vi "Wire RefNum to BBN.vi"(8 "error in (no error)":errorcluster, 9 "Label.Text":string, 10 "Created RefNum":refnum<vi>, 11 "VI in":refnum<vi>) -> (0 "error out":errorcluster)   [LabVIEW 2020]
uses:
  <vilib>/Utility/traverseref.llb/TRef TravTarget.ctl
  <vilib>/Utility/traverseref.llb/VI Scripting - Traverse.lvlib
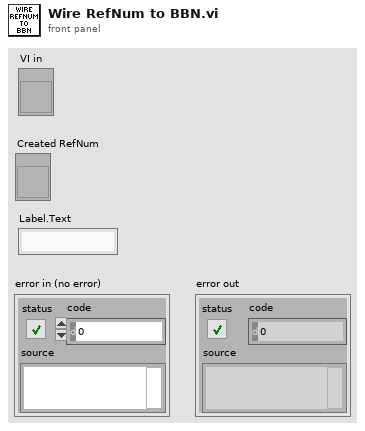
[diagram p1: front panel]
types:
  T1 = typedef "TRef TravTarget.ctl" = enum16{"FP", "BD", "Other"}
  T2 = enum32{"Top Edges", "Vertical Centers", "Bottom Edges", "Vertical Gap", "Vertical Compress", "Left Edges", "Horizontal Centers", "Right Edges", "Horizontal Gap", "Horizontal Compress"}
  T3 = enum32{"Top Edges", "Vertical Centers", "Bottom Edges", "Left Edges", "Horizontal Centers", "Right Edges"}
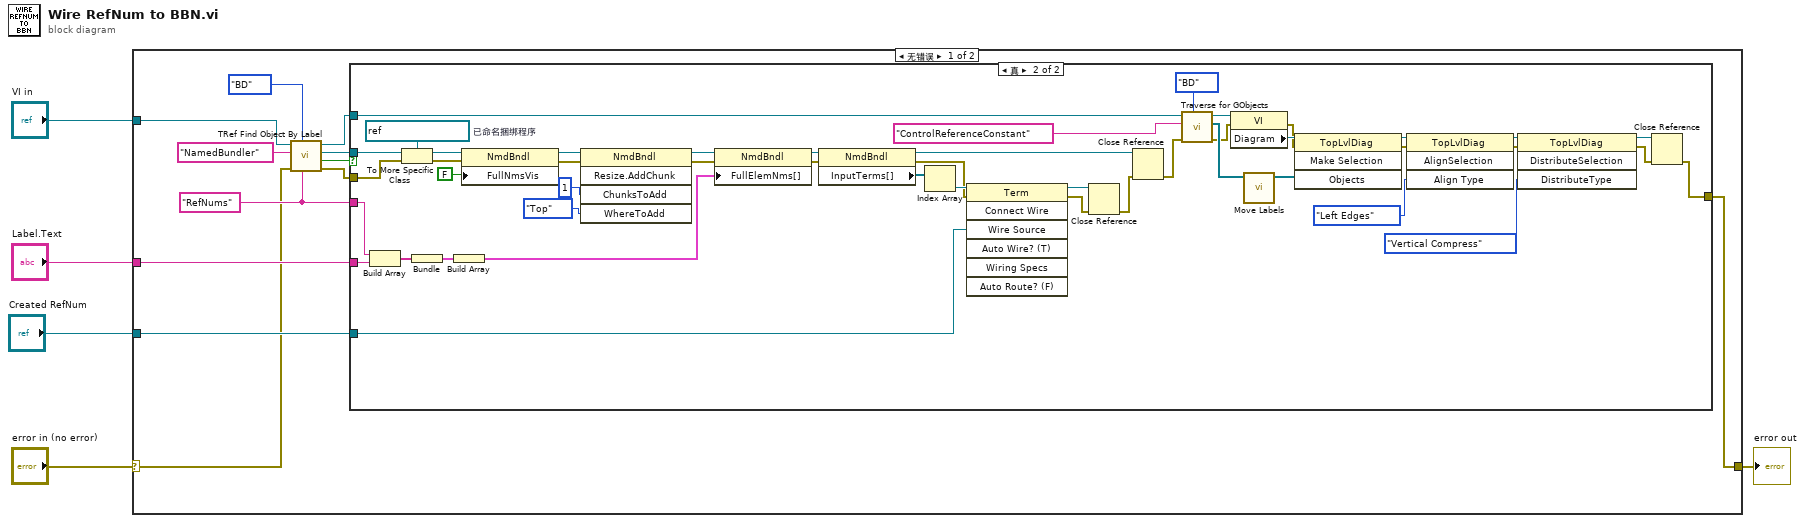
[diagram p0: block diagram]
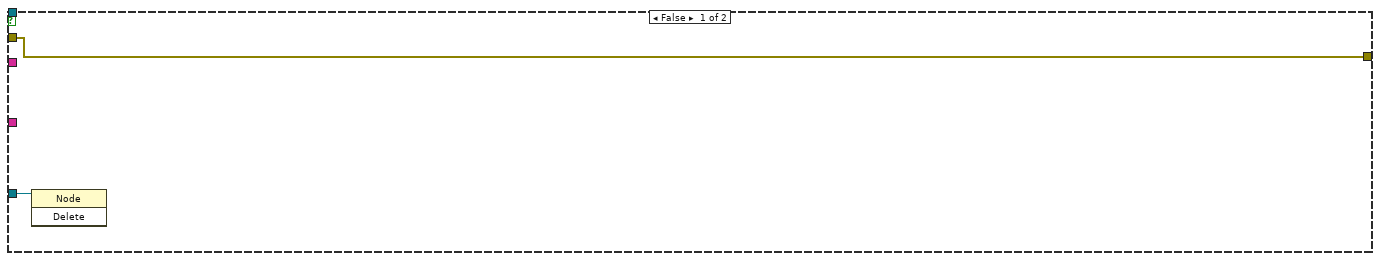
[diagram p2: hidden frame]
diagram:
  n1 = case shown="无错误" "error in (no error)" {
    selector: "error in (no error)" -> [w8 w66]
    tunnel: "Created RefNum" -> [w17 _]
    tunnel: "VI in" -> [w15 _]
    tunnel: "Label.Text" -> [w14 _]
    tunnel: [w6 w66] -> w2
    frame No Error {
      w13 = "RefNums" ("Label.Text")
      n2 = call <vilib>:"TRef Find Object By Label.vi"("Label"=w13, "Traverse Target"=TRef_TravTarget."BD", "error in (no error)"=w8, "Class Name"="NamedBundler", "VI Ref"=w15) -> ("error out"=w7:errorcluster, "Found?"=w12:bool, "Found Obj Ref"=w11:refnum<vi>, "dup VI Ref"=w16:refnum<vi>)  [unwired: 3 in]
      n3 = case shown="真" w12 {
        tunnel: w11 -> [_ w65]
        tunnel: w17 -> [w19 w50]
        tunnel: w14 -> [_ w56]
        tunnel: w13 -> [_ w57]
        tunnel: w16 -> [_ w44]
        tunnel: w7 -> [w18 w38]
        tunnel: [w18 w20] -> w6
        frame False {
          n4 = invoke class="Node" method="Delete"(reference=w19) -> ()  [unwired: 2 in, 3 out]
        }
        frame True {
          w64 = refnum<vi> refnum  # 已命名捆绑程序
          n5 = Build Array(w57, w56) -> (w55:string[])
          n6 = To More Specific Class(target class=w64, reference=w65, error in=w38) -> (specific class reference=w63:refnum<vi>, error out=w37:errorcluster)
          n7 = Bundle(w55) -> (w54:cluster{string[]})  [unwired: 1 in]
          n8 = Build Array(w54) -> (w53:cluster{string[]}[])
          n9 = property class="NmdBndl"(reference=w63, error in=w37, "FullNmsVis"=FALSE ("Full Names Visible?")) -> (reference out=w59:refnum<vi>, error out=w36:errorcluster)
          n10 = invoke class="NmdBndl" method="Resize.AddChunk"(reference=w59, error in=w36, "ChunksToAdd"=u8 1 ("Chunks To Add"), "WhereToAdd"=enum8{"Bottom", "Top"}."Top" ("Where To Add")) -> (reference out=w35:refnum<vi>, error out=w34:errorcluster)  [unwired: 1 in, 3 out]
          n11 = property class="NmdBndl"(reference=w35, error in=w34, "FullElemNms[]"=w53) -> (reference out=w52:refnum<vi>, error out=w33:errorcluster)
          n12 = property class="NmdBndl"(reference=w52, error in=w33) -> (reference out=w23:refnum<vi>, error out=w32:errorcluster, "InputTerms[]"=w58:refnum<vi>[])
          n13 = Index Array(array=w58) -> (element=w51:refnum<vi>)  [unwired: 1 in]
          n14 = invoke class="Term" method="Connect Wire"(reference=w51, error in=w32, "Wire Source"=w50) -> (reference out=w25:refnum<vi>, error out=w24:errorcluster)  [unwired: 4 in, 5 out]
          n15 = Close Reference(reference=w25, error in (no error)=w24) -> (error out=w22:errorcluster)
          n16 = Close Reference(reference=w23, error in (no error)=w22) -> (error out=w21:errorcluster)
          n17 = call <vilib>:"Traverse for GObjects.vi"("Traverse Target"=TRef_TravTarget."BD", "error in (no error)"=w21, "Class Name"="ControlReferenceConstant", "VI Refnum"=w44) -> ("error out"=w31:errorcluster, "References"=w40:refnum<vi>[], "dup VI Refnum"=w42:refnum<vi>)  [unwired: 4 in, 1 out]
          n18 = property class="VI"(reference=w42, error in=w31) -> (error out=w30:errorcluster, "Diagram"=w41:refnum<vi>)  [unwired: 1 out]
          n19 = call "Move Labels.vi"("Objects"=w40) -> ("Objects out"=w39:refnum<vi>[])  [unwired: 9 in, 1 out]
          n20 = invoke on="Invoke Node" class="TopLvlDiag" method="Make Selection"(reference=w41, error in=w30, "Objects"=w39) -> (reference out=w43:refnum<vi>, error out=w29:errorcluster)  [unwired: 1 in, 2 out]
          n21 = invoke on="Invoke Node" class="TopLvlDiag" method="AlignSelection"(reference=w43, error in=w29, "Align Type"=T3."Left Edges") -> (reference out=w48:refnum<vi>, error out=w28:errorcluster)  [unwired: 1 in, 2 out]
          n22 = invoke on="Invoke Node" class="TopLvlDiag" method="DistributeSelection"(reference=w48, error in=w28, "DistributeType"=T2."Vertical Compress") -> (reference out=w27:refnum<vi>, error out=w26:errorcluster)  [unwired: 1 in, 2 out]
          n23 = Close Reference(reference=w27, error in (no error)=w26) -> (error out=w20:errorcluster)
        }
      }
    }
    frame Error {
    }
  }
  "error out" <- w2
